vi "LN_NewNode.vi"(1 "InputContent":i32) -> (0 "OutputListNode":refnum<class "ListNode.lvclass">)   [LabVIEW 2014, in "ListNode.lvclass"]
uses:
  ListNode.lvclass
  ListNode.lvclass/ListNode.ctl
  ListNodeVirtual.lvclass
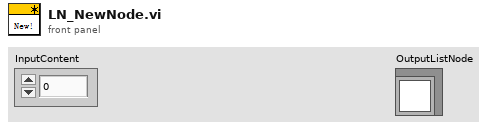
[diagram p1: front panel]
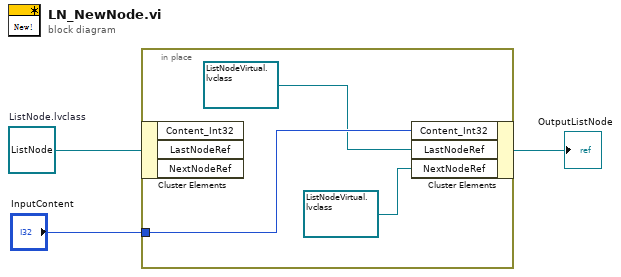
[diagram p0: block diagram]
diagram:
  w3 = refnum<class "ListNode.lvclass"> refnum  # ListNode.lvclass
  n1 = in-place {
    in-place-border: "InputContent" -> [w6]
    n2 = in-place-cluster #1(w3) -> ()  [unwired: 3 out]
    n3 = in-place-cluster #1("Content_Int32"=w6, "LastNodeRef"=refnum<data-value> refnum, "NextNodeRef"=refnum<data-value> refnum) -> (→"OutputListNode":refnum<class "ListNode.lvclass">)
  }
